vi "Create CONNECT Packet.vi"(5 "type":refnum<class "CONNECT.lvclass">, 6 "Keep Alive (s)":u16, 7 "Client ID (empty: generate new)":string, 8 "error in (no error)":errorcluster, 10 "Payload":T1, 11 "Connect Flags":T2) -> (0 "error out":errorcluster, 2 "Bytes Stream":u8[](array[numeric]) format="%08b", 3 "CONNECT":refnum<class "CONNECT.lvclass">)   [LabVIEW 2013, in "MQTT_Control_Packets.lvlib" / "CONNECT.lvclass"]
uses:
  CONNECT.lvclass
  ConnectFlags -- cluster.ctl
  ConnectPayload -- cluster.ctl
  CONNECT.lvclass/CONNECT.ctl
  ControlPacket/ControlPacket.lvclass/ControlPacket.ctl
  ControlPacket/ControlPacket.lvclass
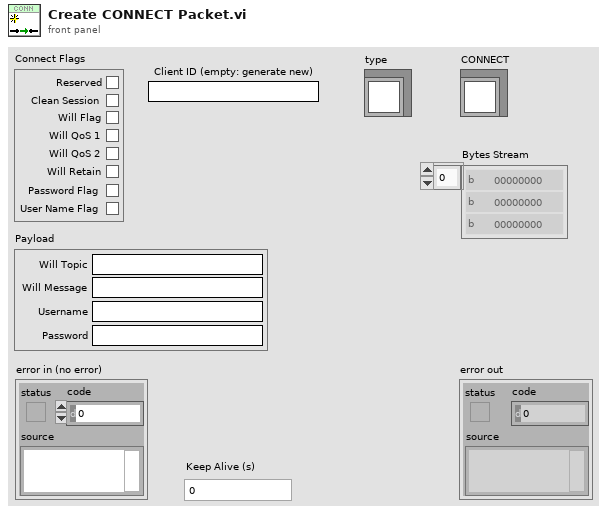
[diagram p1: front panel]
types:
  T1 = typedef "MQTT_Control_Packets.lvlib/CONNECT.lvclass/ConnectPayload -- cluster.ctl" = cluster{"Will Topic":string, "Will Message":string, "Username":string, "Password":string}
  T2 = typedef "MQTT_Control_Packets.lvlib/CONNECT.lvclass/ConnectFlags -- cluster.ctl" = cluster{"Reserved":bool, "Clean Session":bool, "Will Flag":bool, "Will QoS 1":bool, "Will QoS 2":bool, "Will Retain":bool, "Password Flag":bool, "User Name Flag":bool}
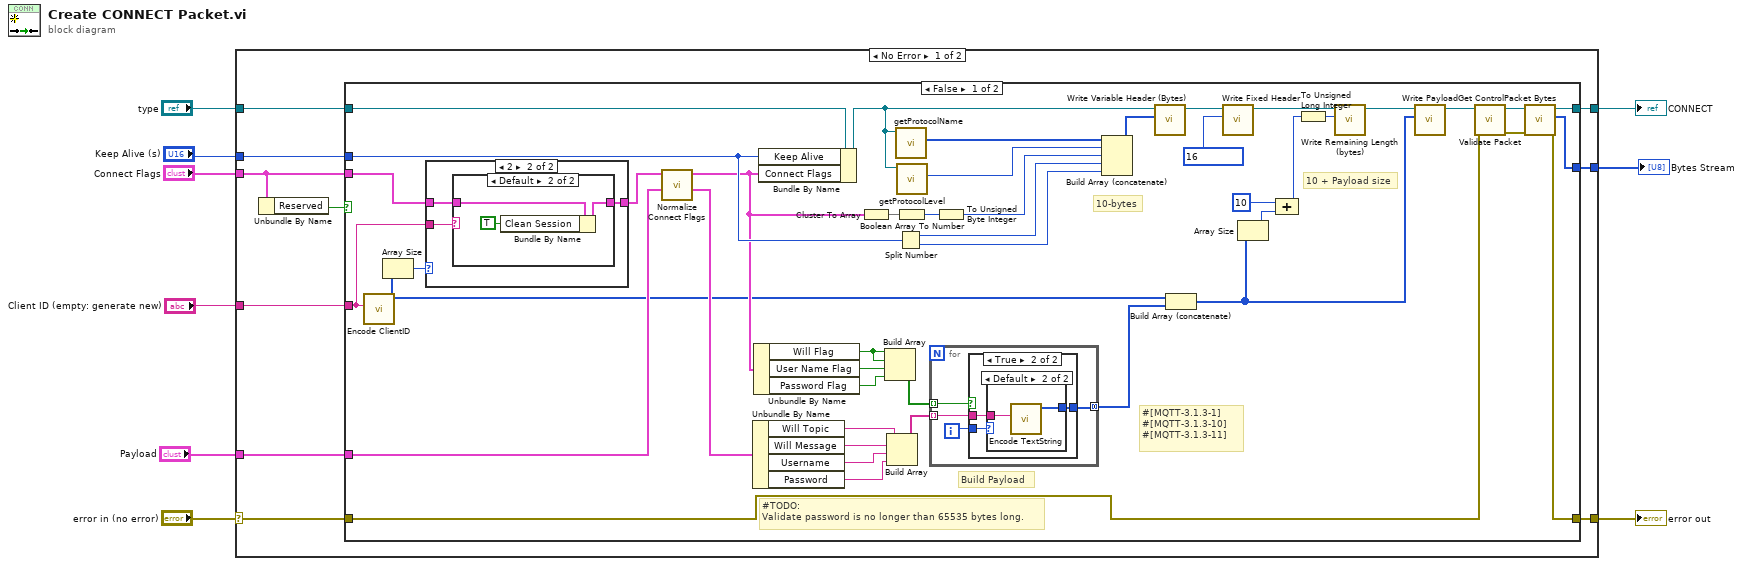
[diagram p0: block diagram]
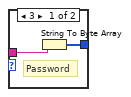
[diagram p5: hidden frame]
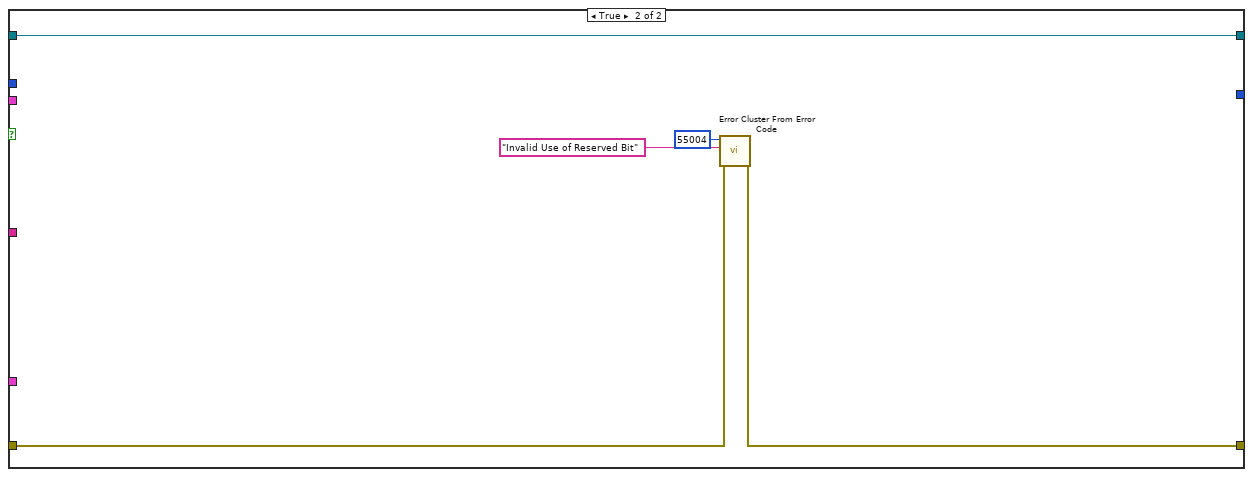
[diagram p6: hidden frame]
diagram:
  n1 = case shown="No Error" "error in (no error)" {
    selector: "error in (no error)" -> [w17 w90]
    tunnel: [w18 w90] -> w8
    tunnel: [w15 w89] -> w6
    tunnel: "type" -> [w16 w89]
    tunnel: "Connect Flags" -> [w14 _]
    tunnel: "Keep Alive (s)" -> [w13 _]
    tunnel: "Client ID (empty: generate new)" -> [w12 _]
    tunnel: "Payload" -> [w11 _]
    tunnel: [w10 _] -> w1
    frame No Error {
      n2 = Unbundle By Name(w14) -> ("Reserved"=w19:bool)
      n3 = case shown="False" w19 {
        tunnel: [w21 w86] -> w18
        tunnel: w17 -> [w33 w85]
        tunnel: w16 -> [w64 w84]
        tunnel: [w23 w84] -> w15
        tunnel: w14 -> [w27 _]
        tunnel: w13 -> [w57 _]
        tunnel: w12 -> [w25 _]
        tunnel: w11 -> [w31 _]
        tunnel: [w20 _] -> w10
        frame False {
          # "Build Payload"
          # "#TODO: \nValidate password is no longer than 65535 bytes long."
          # "#[MQTT-3.1.3-1]\n#[MQTT-3.1.3-10]\n#[MQTT-3.1.3-11]"
          # "10-bytes"
          # "10 + Payload size"
          n4 = call "Encode ClientID.vi"("Client ID (empty: generate new)"=w25) -> ("Length-Prefixed Field"=w29:u8[])  [unwired: 9 in, 1 out]
          n5 = Array Size(array=w29) -> (size(s)=w28:i32)
          n6 = case shown="2" w28 {
            tunnel: w27 -> [w65 w68]
            tunnel: [w65 w67] -> w26
            tunnel: w25 -> [_ w66]
            frame Default {
            }
            frame 2 {
              n7 = case shown="Default" w66 {
                tunnel: w68 -> [w69 w72]
                tunnel: [w69 w71] -> w67
                frame "%%EMPTY%%" {
                }
                frame Default {
                  n8 = Bundle By Name(cluster=w72, "Clean Session"=TRUE) -> (w71:T2)
                }
              }
            }
          }
          n9 = call "Normalize Connect Flags.vi"("Payload"=w31, "Connect Flags in"=w26) -> ("Payload out"=w30:T1, "Connect Flags out"=w32:T2)  [unwired: 8 in]
          n10 = Unbundle By Name(w30) -> ("Will Topic"=w44:string, "Will Message"=w43:string, "Username"=w42:string, "Password"=w41:string)
          n11 = Unbundle By Name(w32) -> ("Will Flag"=w47:bool, "User Name Flag"=w46:bool, "Password Flag"=w45:bool)
          n12 = Bundle By Name(cluster=w64, "Keep Alive"=w57, "Connect Flags"=w32) -> (w56:refnum<class "CONNECT.lvclass">)
          n13 = Cluster To Array(cluster=w32) -> (array=w63:bool[])
          n14 = Build Array(w47, w47, w46, w45) -> (w40:bool[])
          n15 = Build Array(w44, w43, w42, w41) -> (w39:string[])
          n16 = call "getProtocolName.vi"("CONNECT in"=w56) -> ("ProtocolName"=w62:u8[])  [unwired: 9 in, 1 out]
          n17 = Split Number(x=w57) -> (hi(x)=w37:u8, lo(x)=w36:u8)
          n18 = call-dynamic "getProtocolLevel.vi"("CONNECT in"=w56) -> ("Protocol Level"=w61:u8)  [unwired: 9 in, 1 out]
          n19 = Boolean Array To Number(Boolean array=w63) -> (number=w60:u32)
          n20 = for {
            tunnel: w40 -> [w76] mode=indexing
            tunnel: w39 -> [w75] mode=indexing
            tunnel: [w74] -> w38 mode=concatenating
            i -> [w73]
            n21 = case shown="True" w76 {
              tunnel: w75 -> [_ w79]
              tunnel: [_ w78] -> w74
              tunnel: w73 -> [_ w77]
              frame False {
              }
              frame True {
                n22 = case shown="Default" w77 {
                  tunnel: w79 -> [w80 w83]
                  tunnel: [w81 w82] -> w78
                  frame 3 {
                    # "Password"
                    n23 = String To Byte Array(string=w80) -> (unsigned byte array=w81:u8[])
                  }
                  frame Default {
                    n24 = call "Encode TextString.vi"("Text String"=w83) -> ("Length-Prefixed Field"=w82:u8[])  [unwired: 10 in]
                  }
                }
              }
            }
          }
          n25 = To Unsigned Byte Integer(number=w60) -> (unsigned 8bit integer=w59:u8)
          n26 = Build Array (concatenate)(w62, w61, w59, w37, w36) -> (w58:u8[])
          n27 = call "Write Variable Header (Bytes).vi"("Variable Header (Bytes)"=w58, "ControlPacket in"=w56) -> ("ControlPacket out"=w55:refnum<class "CONNECT.lvclass">)  [unwired: 9 in]
          n28 = Build Array (concatenate)(w29, w38) -> (w35:u8[])
          n29 = call "Write Fixed Header.vi"("Fixed Header"=u8 16, "ControlPacket in"=w55) -> ("ControlPacket out"=w53:refnum<class "CONNECT.lvclass">)  [unwired: 9 in]
          n30 = Array Size(array=w35) -> (size(s)=w51:i32)
          n31 = Compound Arithmetic op=ADD(10 ("value"), w51) -> (w49:i32)
          n32 = To Unsigned Long Integer(number=w49) -> (unsigned 32bit integer=w48:u32)
          n33 = call "Write Remaining Length (bytes).vi"("Remaining Length (bytes)"=w48, "ControlPacket in"=w53) -> ("ControlPacket out"=w52:refnum<class "CONNECT.lvclass">)  [unwired: 9 in]
          n34 = call "Write Payload.vi"("Payload"=w35, "ControlPacket in"=w52) -> ("ControlPacket out"=w34:refnum<class "CONNECT.lvclass">)  [unwired: 9 in]
          n35 = call "Validate Packet.vi"("error in (no error)"=w33, "ControlPacket in"=w34) -> ("error out"=w22:errorcluster, "ControlPacket out"=w24:refnum<class "CONNECT.lvclass">)  [unwired: 8 in]
          n36 = call "Get ControlPacket Bytes.vi"("error in (no error)"=w22, "ControlPacket"=w24) -> ("error out"=w21:errorcluster, "Bytes Stream"=w20:u8[], "ControlPacket dup"=w23:refnum<class "CONNECT.lvclass">)  [unwired: 6 in, 1 out]
        }
        frame True {
          n37 = call <vilib>:"Error Cluster From Error Code.vi"("error in (no error)"=w85, "error message (\"\")"="Invalid Use of Reserved Bit" ("error message (\"\")"), "error code (0)"=55004) -> ("error out"=w86:errorcluster)  [unwired: 6 in]
        }
      }
    }
    frame Error {
    }
  }
  "error out" <- w8
  "CONNECT" <- w6
  "Bytes Stream" <- w1
